vi "create raster triangle.vi"() -> ()   [LabVIEW 2009]
panel:
  in  "index offset":i32
  out "map":bool[][](array[boolean])
  out "rectangle":T1
  in  "object":T2 {"direction" step=0.1}
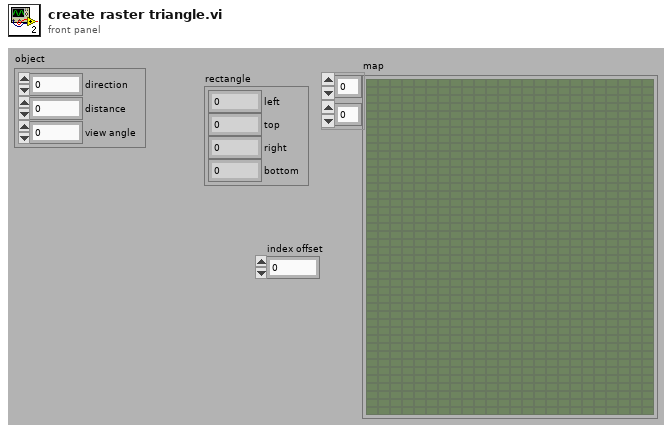
[diagram p1: front panel]
types:
  T1 = cluster{"left":i16, "top":i16, "right":i16, "bottom":i16}
  T2 = cluster{"direction":dbl, "distance":i32, "view angle":dbl}
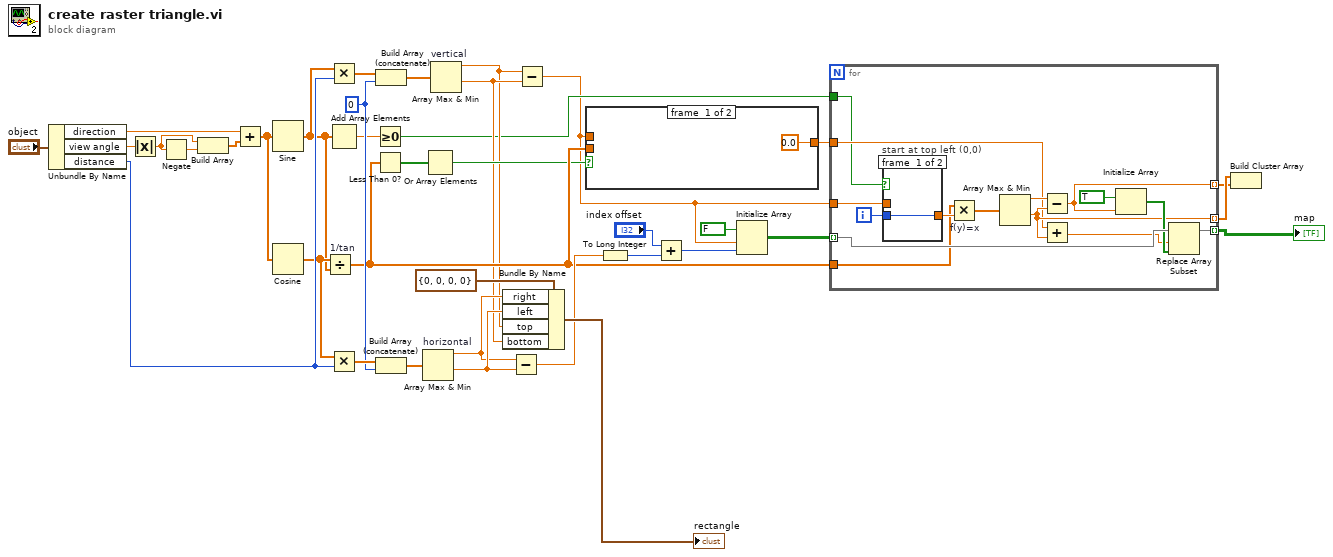
[diagram p0: block diagram]
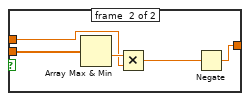
[diagram p2: hidden frame]
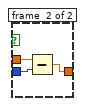
[diagram p3: hidden frame]
diagram:
  w25 = 0
  n1 = Unbundle By Name("object") -> ("direction"=w31:dbl, "view angle"=w33:dbl, "distance"=w18:i32)
  n2 = Absolute Value(x=w33) -> (abs(x)=w29:dbl)
  n3 = Negate(x=w29) -> (-x=w34:dbl)
  n4 = Build Array(w29, w34) -> (w32:dbl[])
  n5 = Add(x=w31, y=w32) -> (x+y=w30:dbl[])
  n6 = Sine(x=w30) -> (sin(x)=w6:dbl[])
  n7 = Cosine(x=w30) -> (cos(x)=w16:dbl[])
  n8 = Divide "1/tan"(x=w16, y=w6) -> (x/y=w9:dbl[])
  n9 = Multiply(x=w6, y=w18) -> (x*y=w27:dbl[])
  n10 = Add Array Elements(numeric array=w6) -> (sum=w5:dbl)
  n11 = Multiply(x=w16, y=w18) -> (x*y=w26:dbl[])
  n12 = Greater Or Equal To 0?(x=w5) -> (x >= 0?=w2:bool)
  n13 = Less Than 0?(x=w9) -> (x < 0?=w10:bool[])
  n14 = Build Array (concatenate)(w27, w25) -> (w24:dbl[])
  n15 = Build Array (concatenate)(w26, w25) -> (w23:dbl[])
  n16 = Array Max & Min "horizontal"(array=w23) -> (max value=w20:dbl, min value=w21:dbl)  [unwired: 2 out]
  n17 = Or Array Elements(Boolean array=w10) -> (logical OR=w7:bool)
  n18 = Array Max & Min "vertical"(array=w24) -> (max value=w3:dbl, min value=w4:dbl)  [unwired: 2 out]
  n19 = Bundle By Name(cluster=T1 {"left"=0, "top"=0, "right"=0, "bottom"=0} ("rect"), "right"=w20, "left"=w21, "top"=w3, "bottom"=w4) -> (→"rectangle":T1)
  n20 = Subtract(x=w20, y=w21) -> (x-y=w19:dbl)
  n21 = Subtract(x=w3, y=w4) -> (x-y=w1:dbl)
  n22 = case shown="True" w7 {
    tunnel: w9 -> [_ w43]
    tunnel: w1 -> [_ w41]
    tunnel: [0.0 w39] -> w8
    frame #0 {
    }
    frame #1 {
      n23 = Array Max & Min(array=w43) -> (min value=w42:dbl)  [unwired: 3 out]
      n24 = Multiply(x=w42, y=w41) -> (x*y=w40:dbl)
      n25 = Negate(x=w40) -> (-x=w39:dbl)
    }
  }
  n26 = To Long Integer(number=w19) -> (32bit integer=w12:i32)
  n27 = Add(x="index offset", y=w12) -> (x+y=w11:i32)
  n28 = Initialize Array(FALSE, w1, w11) -> (w17:bool[][])
  n29 = for {
    tunnel: w17 -> [w58] mode=indexing
    tunnel: w1 -> [w54]
    tunnel: w9 -> [w52]
    tunnel: [w49] -> w35 mode=indexing
    tunnel: [w47] -> w15 mode=indexing
    tunnel: [w48] -> w14 mode=indexing
    tunnel: w8 -> [w46]
    tunnel: w2 -> [w44]
    i -> [w55]
    n30 = case "start at top left (0,0)" shown="False" w44 {
      tunnel: w55 -> [w59 w62]
      tunnel: w54 -> [_ w61]
      tunnel: [w59 w60] -> w53
      frame #0 {
      }
      frame #1 {
        n31 = Subtract(x=w61, y=w62) -> (x-y=w60:dbl)
      }
    }
    n32 = Multiply "f(y)=x"(x=w52, y=w53) -> (x*y=w51:dbl[])
    n33 = Array Max & Min(array=w51) -> (max value=w50:dbl, min value=w47:dbl)  [unwired: 2 out]
    n34 = Subtract(x=w50, y=w47) -> (x-y=w48:dbl)
    n35 = Add(x=w46, y=w47) -> (x+y=w45:dbl)
    n36 = Initialize Array(TRUE, w48) -> (w57:bool[])
    n37 = Replace Array Subset(array=w58, new element=w57, index=w45) -> (w49:bool[])
  }
  "map" <- w35
  n38 = Build Cluster Array(w15, w14) -> ()  [unwired: 1 out]
